vi "Acnet XML-RPC Device Reader.vi"(8 "error in (no error)":errorcluster, 11 "Device":string) -> (0 "error out":errorcluster, 3 "Reading":T1)   [LabVIEW 2013]
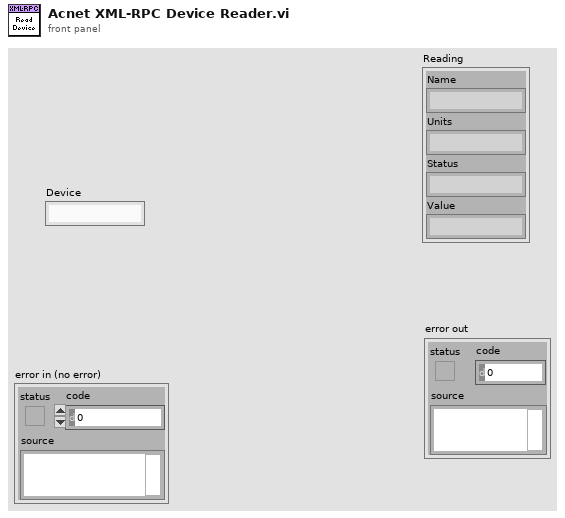
[diagram p1: front panel]
types:
  T1 = cluster{"Name":string, "Units":string, "Status":string, "Value":string}
  T2 = cluster{"Name":string, "Units":string, "Status":string, "Value":string}[]
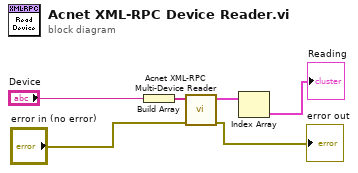
[diagram p0: block diagram]
diagram:
  n1 = Build Array("Device") -> (w5:string[])
  n2 = call "Acnet XML-RPC Multi-Device Reader.vi"("error in (no error)"="error in (no error)", "Devices"=w5) -> ("error out"=→"error out":errorcluster, "Readings"=w2:T2)  [unwired: 8 in]
  n3 = Index Array(array=w2) -> (element=→"Reading":T1)  [unwired: 1 in]
